vi "Example_LDA.vi"() -> ()   [LabVIEW 2009]
uses:
  <vilib>/Utility/miscctls.llb/LV3DPointTypeDef.ctl
  <vilib>/addons/Machine Learning/Visualization/Visualization (2D).vi
  <vilib>/addons/Machine Learning/Visualization/Visualization (3D).vi
  <vilib>/addons/Machine Learning/NILabs_MLT.lvlib
  <vilib>/picture/3D Picture Control/NI_3D Picture Control.lvlib
panel:
  out "2-D Projection of the data":cluster{"X":dbl[], "Y":dbl[]}[](graph)
  out "w":dbl[][](array[numeric])
  in  "# of samples":i32=1024
  out "3-D data":refnum<vi>(3d-picture)
  # "Introduction:\nLinear Discriminant Analysis (LDA) is used to project a 3-D data to a 2-D space, while preserving as much of the class discriminatory information as possible.\nw indicates the resulting directions to project the data. Each colomn of w represents one direction."
  # "(Samples are overlain with class labels.)"
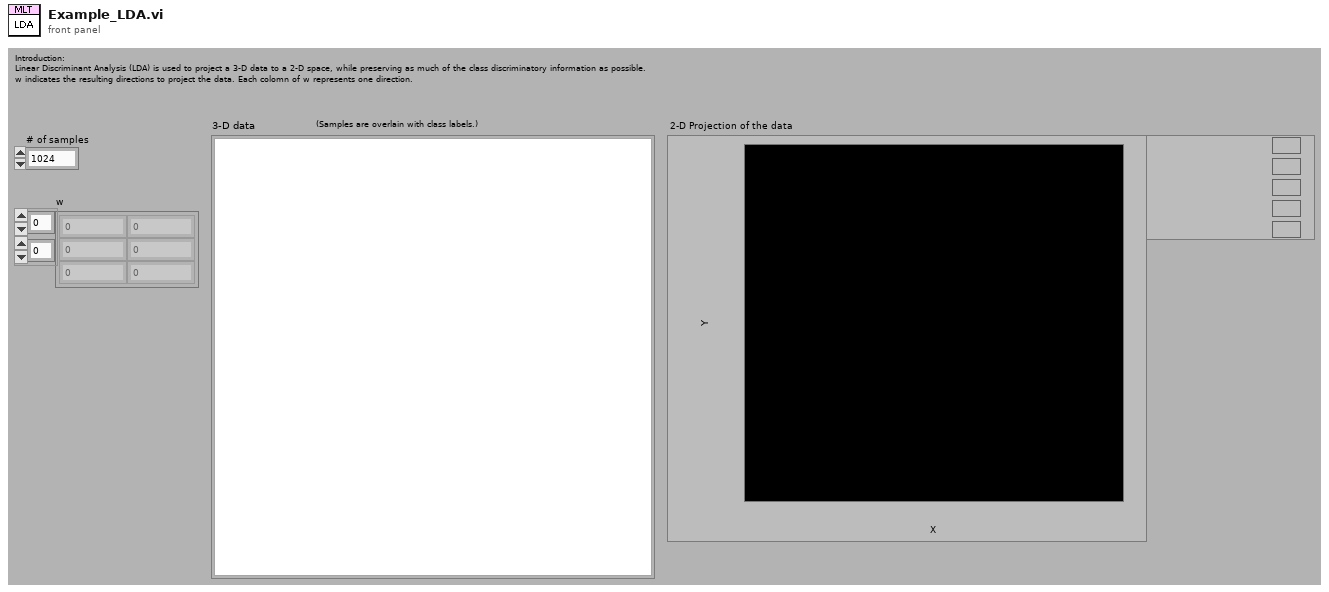
[diagram p1: front panel]
types:
  T1 = enum16{"Overall", "Per Primitive", "Per Vertex", "Binding Off"}
  T2 = enum16{"Points", "Lines", "Line Strip", "Line Loop", "Triangles", "Triangle Strip", "Triangle Fan", "Quads", "Quad Strip", "Polygon"}
  T3 = typedef "LV3DPointTypeDef.ctl" = cluster{"X":sgl, "Y":sgl, "Z":sgl}
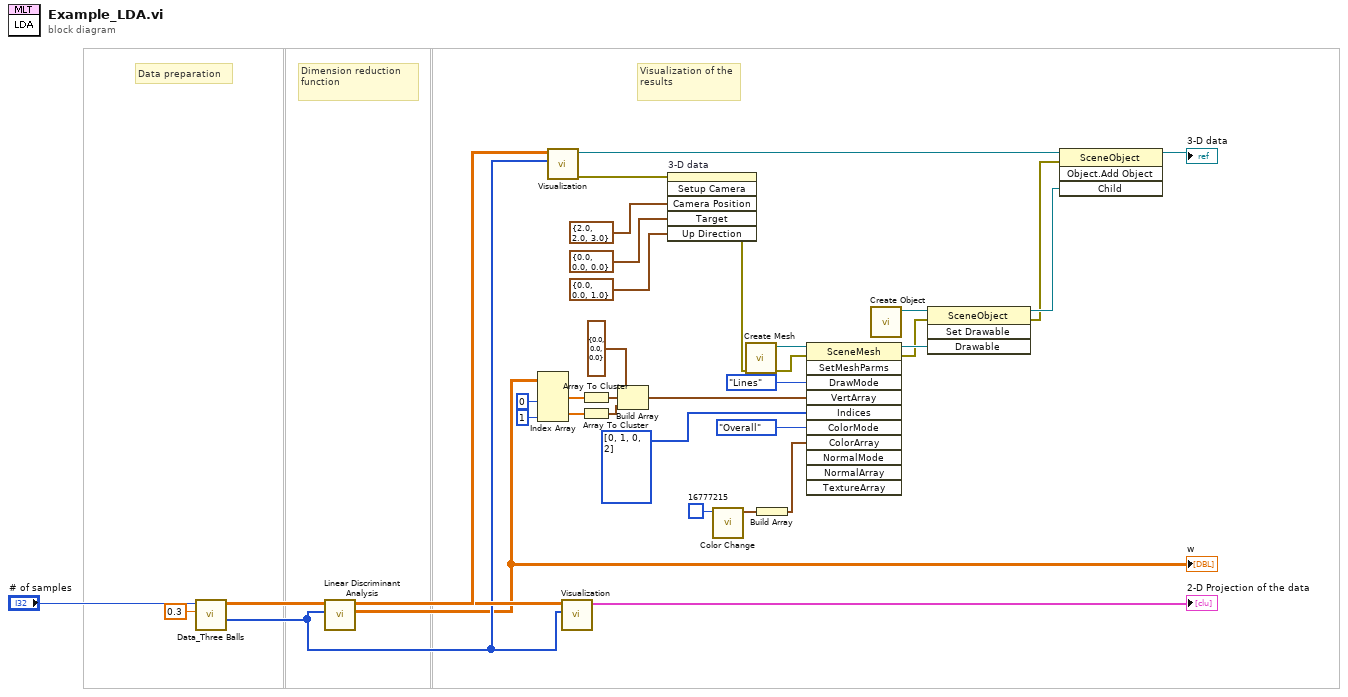
[diagram p0: block diagram]
diagram:
  # "Visualization of the results"
  # "Dimension reduction function"
  # "Data preparation"
  n1 = call "Data_Three Balls.vi"("noise amplitude"=0.3, "# of points"="# of samples") -> ("Classes"=w27:i32[], "Data"=w29:dbl[][])  [unwired: 8 in]
  n2 = call <vilib>:"Linear Discriminant Analysis.vi"("Class labels"=w27, "Examples"=w29) -> ("w"=w15:dbl[][], "Projected Examples"=w28:dbl[][])  [unwired: 7 in, 1 out]
  "w" <- w15
  n3 = Index Array(array=w15, index (col) #1=0 ("disabled index (col)"), index (col) #2=1 ("index (col)")) -> (element #1=w12:dbl[], element #2=w11:dbl[])  [unwired: 2 in]
  n4 = call-poly <vilib>:"Visualization.vi"("Class labels"=w27, "Data samples"=w29) -> ("error out"=w31:errorcluster, "3D Picture"=w5:refnum<vi>)  [unwired: 8 in]
  n5 = call-poly <vilib>:"Visualization.vi"("Class labels"=w27, "Data samples"=w28) -> ("XY Graph"=→"2-D Projection of the data":cluster{"X":dbl[], "Y":dbl[]}[])  [unwired: 8 in, 1 out]
  n6 = Array To Cluster(array=w12) -> (cluster=w9:cluster{"w[0]":dbl, "w[1]":dbl, "w[2]":dbl})
  n7 = Array To Cluster(array=w11) -> (cluster=w10:cluster{"w[0]":dbl, "w[1]":dbl, "w[2]":dbl})
  n8 = Build Array(cluster{"w[0]":dbl, "w[1]":dbl, "w[2]":dbl} {"w[0]"=0.0, "w[1]"=0.0, "w[2]"=0.0} ("element"), w9, w10) -> (w7:cluster{"w[0]":dbl, "w[1]":dbl, "w[2]":dbl}[])
  n9 = invoke on="3-D data" class="SceneGraphDisp (strict)" method="Setup Camera"(error in=w31, "Camera Position"=T3 {"X"=2.0, "Y"=2.0, "Z"=3.0}, "Target"=T3 {"X"=0.0, "Y"=0.0, "Z"=0.0} ("Camera Position"), "Up Direction"=T3 {"X"=0.0, "Y"=0.0, "Z"=1.0} ("Camera Position")) -> (error out=w2:errorcluster)  [unwired: 2 in, 5 out]
  n10 = call <vilib>:"Color Change.vi"("Color"=u32 16777215) -> ("RGBA"=w17:cluster{"R":sgl, "G":sgl, "B":sgl, "A":sgl})  [unwired: 10 in]
  n11 = call <vilib>:"Create Mesh.vi"("error in (no error)"=w2) -> ("error out"=w20:errorcluster, "New Mesh Refnum"=w25:refnum<vi>)  [unwired: 9 out]
  n12 = Build Array(w17) -> (w16:cluster{"R":sgl, "G":sgl, "B":sgl, "A":sgl}[])
  n13 = invoke class="SceneMesh" method="SetMeshParms"(reference=w25, error in=w20, "DrawMode"=T2."Lines" ("Draw Mode"), "VertArray"=w7, "Indices"=u32[] [0, 1, 0, 2], "ColorMode"=T1."Overall" ("Color Binding Mode"), "ColorArray"=w16) -> (reference out=w23:refnum<vi>, error out=w21:errorcluster)  [unwired: 4 in, 9 out]
  n14 = call <vilib>:"Create Object.vi"() -> ("Scene:New Object"=w24:refnum<vi>)  [unwired: 2 in, 9 out]
  n15 = invoke class="SceneObject" method="Set Drawable"(reference=w24, error in=w21, "Drawable"=w23) -> (reference out=w3:refnum<vi>, error out=w1:errorcluster)  [unwired: 1 in, 2 out]
  n16 = invoke class="SceneObject" method="Object.Add Object"(reference=w5, error in=w1, "Child"=w3) -> (reference out=→"3-D data":refnum<vi>)  [unwired: 1 in, 3 out]
